vi "_11_Sample_qsns_03[14].vi"() -> ()   [LabVIEW 2020]
panel:
  out "initialized array":dbl[](array[numeric])
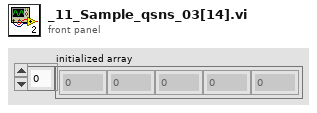
[diagram p1: front panel]
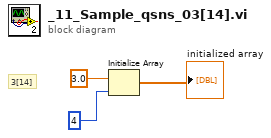
[diagram p0: block diagram]
diagram:
  # "3[14]"
  n1 = Initialize Array "Initialize Array"(3.0 ("element"), 4) -> (→"initialized array":dbl[])
